vi "Get Vi Reference.vi"(7 "error in (no error)":errorcluster, 9 "Control name":string, 10 "Vi Reference in":refnum<vi>) -> (0 "error out":errorcluster, 2 "控件值:获取全部":cluster{"Name":string, "Variant Data":variant}[](array[cluster]), 3 "队列输出":refnum<queue>)   [LabVIEW 2016]
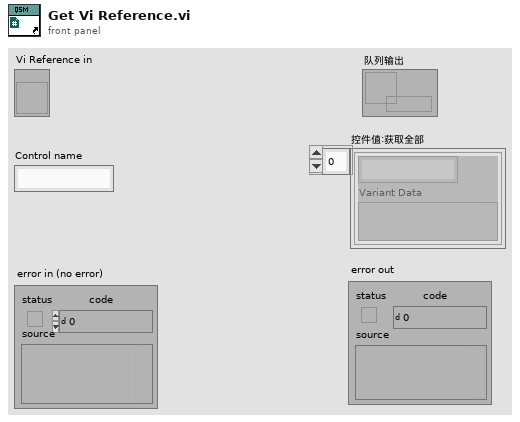
[diagram p1: front panel]
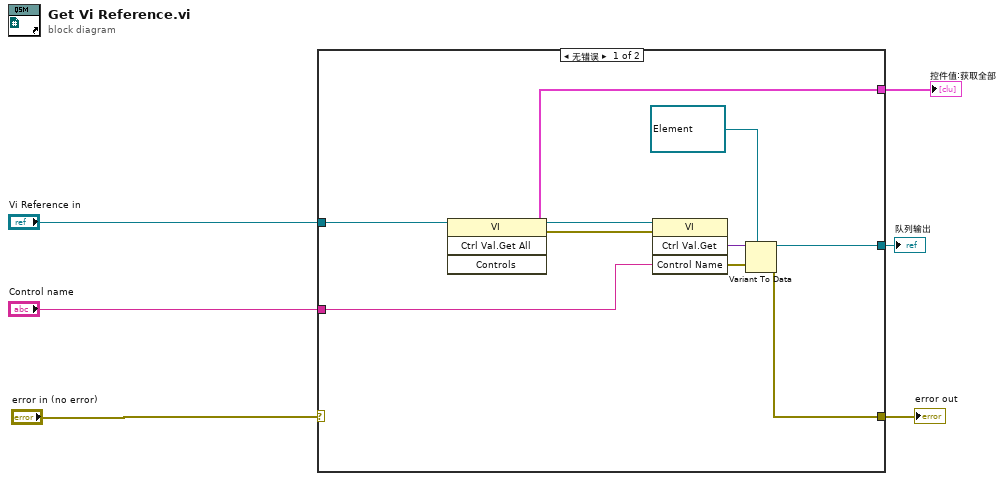
[diagram p0: block diagram]
diagram:
  n1 = case shown="无错误" "error in (no error)" {
    selector: "error in (no error)" -> [_ w17]
    tunnel: "Vi Reference in" -> [w7 _]
    tunnel: "Control name" -> [w15 _]
    tunnel: [w9 w17] -> w4
    tunnel: [w13 _] -> w3
    tunnel: [w10 _] -> w1
    frame No Error {
      n2 = invoke class="VI" method="Ctrl Val.Get All"(reference=w7) -> (reference out=w16:refnum<vi>, error out=w14:errorcluster, "Get All Control Values Variant"=w13:cluster{"Name":string, "Variant Data":variant}[])  [unwired: 3 in, 1 out]
      n3 = invoke class="VI" method="Ctrl Val.Get"(reference=w16, error in=w14, "Control Name"=w15) -> (error out=w8:errorcluster, "Get Control Value Variant"=w12:variant)  [unwired: 1 in, 2 out]
      n4 = Variant To Data(error in=w8, type=refnum<queue> refnum, Variant=w12) -> (data=w10:refnum<queue>, error out=w9:errorcluster)
    }
    frame Error {
    }
  }
  "error out" <- w4
  "控件值:获取全部" <- w3
  "队列输出" <- w1
